vi "Control bars.vi"() -> ()   [LabVIEW 2012]
uses:
  Bar info.ctl
panel:
  in  "Go":bool
  in  "Quit":bool
  in  "Refresh rate":dbl
  in  "Bar width":dbl=2.0
  in  "Bar speed":dbl=10.0
  in  "Monitor scale":dbl=40.0
  in  "Amplitude":dbl
  in  "Frequency":dbl
  in  "Contrast":dbl=1.0
  # "cm"
  # "cm/sec"
  # "cm/sec"
  # "Hz"
  # "Hz"
  # "pix/cm"
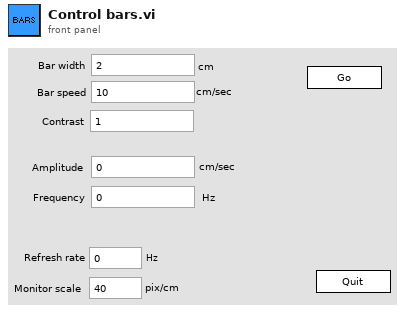
[diagram p1: front panel]
types:
  T1 = typedef "Bar info.ctl" = cluster{"Bar width":dbl, "Bar speed":dbl, "Amplitude":dbl, "Frequency":dbl, "Contrast":dbl, "Refresh rate":dbl, "Monitor scale":dbl, "Command":enum16{"Go", "Stop"}}
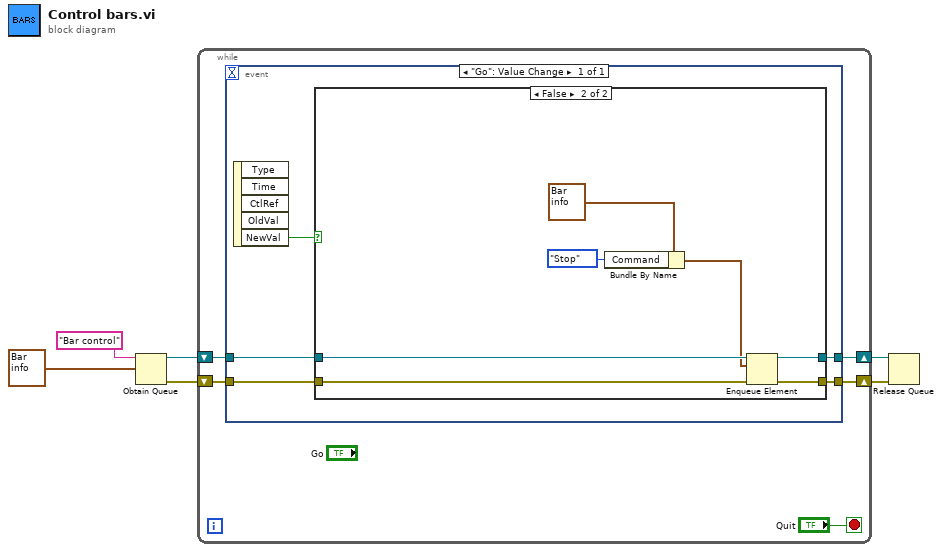
[diagram p0: block diagram]
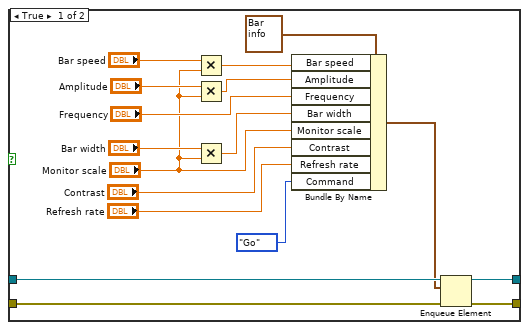
[diagram p2: hidden frame]
diagram:
  n1 = Obtain Queue(name (unnamed)="Bar control", element data type=T1 {"Bar width"=2.0, "Bar speed"=10.0, "Amplitude"=0.0, "Frequency"=0.0, "Contrast"=1.0, "Refresh rate"=0.0, "Monitor scale"=40.0, "Command"=enum."Stop"} ("Bar info")) -> (queue out=w4:refnum<queue>, error out=w3:errorcluster)  [unwired: 3 in, 1 out]
  n2 = while {
    shift-right: [w8] -> w2
    shift-left: w3 -> [w9]
    shift-right: [w7] -> w1
    shift-left: w4 -> [w10]
    stop <- "Quit" stop-if-true
    n3 = event shown="[0] \"Go\": Value Change" {
      selector: _ -> [_]
      dyn-events: _ -> [_]
      timeout: _ -> [_]
      tunnel: w10 -> [w15]
      tunnel: w9 -> [w14]
      tunnel: [w13] -> w8
      tunnel: [w12] -> w7
      event "Go": Value Change {
        n4 = event-data() -> ("NewVal"=w16:bool)  [unwired: 1 in, 4 out]
        n5 = case shown="False" w16 {
          tunnel: w15 -> [w21 w38]
          tunnel: w14 -> [w19 w36]
          tunnel: [w18 w35] -> w13
          tunnel: [w17 w34] -> w12
          frame True {
            n6 = Multiply(x="Bar speed", y="Monitor scale") -> (x*y=w30:dbl)
            n7 = Multiply(x="Amplitude", y="Monitor scale") -> (x*y=w29:dbl)
            n8 = Multiply(x="Bar width", y="Monitor scale") -> (x*y=w27:dbl)
            n9 = Bundle By Name(cluster=T1 {"Bar width"=2.0, "Bar speed"=10.0, "Amplitude"=0.0, "Frequency"=0.0, "Contrast"=1.0, "Refresh rate"=0.0, "Monitor scale"=40.0, "Command"=enum."Stop"} ("Bar info"), "Bar speed"=w30, "Amplitude"=w29, "Frequency"="Frequency", "Bar width"=w27, "Monitor scale"="Monitor scale", "Contrast"="Contrast", "Refresh rate"="Refresh rate", "Command"=enum16{"Go", "Stop"}."Go") -> (w20:T1)
            n10 = Enqueue Element(queue=w21, element=w20, error in (no error)=w19) -> (queue out=w17:refnum<queue>, error out=w18:errorcluster)  [unwired: 1 in, 1 out]
          }
          frame False {
            n11 = Bundle By Name(cluster=T1 {"Bar width"=2.0, "Bar speed"=10.0, "Amplitude"=0.0, "Frequency"=0.0, "Contrast"=1.0, "Refresh rate"=0.0, "Monitor scale"=40.0, "Command"=enum."Stop"} ("Bar info"), "Command"=enum16{"Go", "Stop"}."Stop") -> (w37:T1)
            n12 = Enqueue Element(queue=w38, element=w37, error in (no error)=w36) -> (queue out=w34:refnum<queue>, error out=w35:errorcluster)  [unwired: 1 in, 1 out]
          }
        }
      }
    }
  }
  n13 = Release Queue(queue=w1, error in (no error)=w2) -> ()  [unwired: 1 in, 3 out]
